vi "Make.vi"(8 "error in (no error)":errorcluster, 11 "Electrical in":refnum<class "BlackElectrical.lvclass">) -> (0 "error out":errorcluster, 3 "Electrical out":refnum<class "BlackElectrical.lvclass">)   [LabVIEW 2014, in "BlackElectrical.lvclass"]
uses:
  BlackElectrical.lvclass
  Electrical/Electrical.lvclass
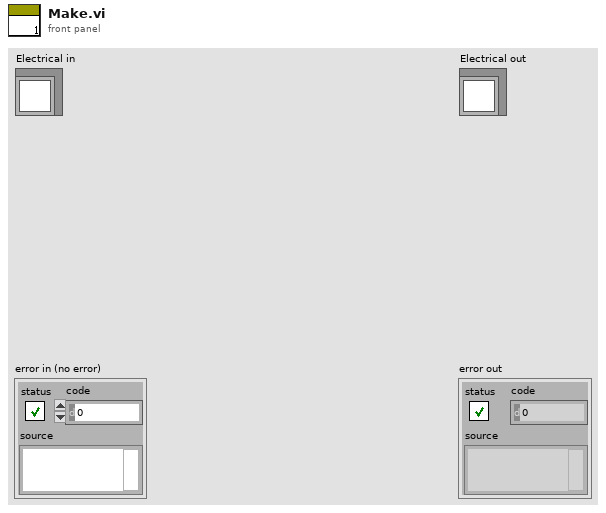
[diagram p1: front panel]
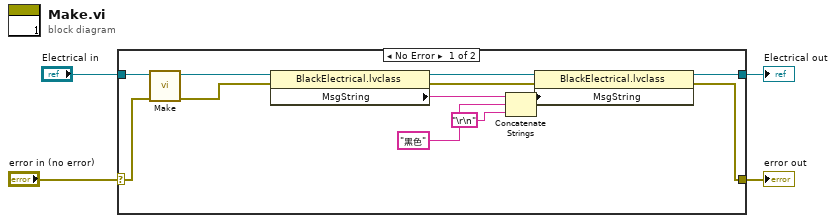
[diagram p0: block diagram]
diagram:
  n1 = case shown="No Error" "error in (no error)" {
    selector: "error in (no error)" -> [w16 w18]
    tunnel: [w14 w18] -> w4
    tunnel: [w12 w17] -> w3
    tunnel: "Electrical in" -> [w6 w17]
    frame No Error {
      n2 = call-parent "Make.vi"("error in (no error)"=w16, "Electrical in"=w6) -> ("error out"=w7:errorcluster, "Electrical out"=w5:refnum<class "BlackElectrical.lvclass">)  [unwired: 8 in]
      n3 = property class="BlackElectrical.lvclass"(reference=w5, error in=w7) -> (reference out=w13:refnum<class "BlackElectrical.lvclass">, error out=w15:errorcluster, "MsgString"=w11:string)
      n4 = Concatenate Strings(w11, "黑色", "\r\n") -> (w10:string)
      n5 = property class="BlackElectrical.lvclass"(reference=w13, error in=w15, "MsgString"=w10) -> (reference out=w12:refnum<class "BlackElectrical.lvclass">, error out=w14:errorcluster)
    }
    frame Error {
    }
  }
  "error out" <- w4
  "Electrical out" <- w3
